vi "SetTilesTMX.vi"(8 "error in (no error)":errorcluster, 9 "Position":T1, 10 "path to tmx-file (created with Tiles2D)":path=path "/home/lvuser/natinst/bin/data/maps/Menu.tmx", 11 "Game in":refnum<class "Game.lvclass">) -> (0 "error out":errorcluster, 3 "Game out":refnum<class "Game.lvclass">)   [LabVIEW 2019, in "RT_Game.lvlib" / "Game.lvclass"]
uses:
  Game.lvclass
  Coordinate.ctl
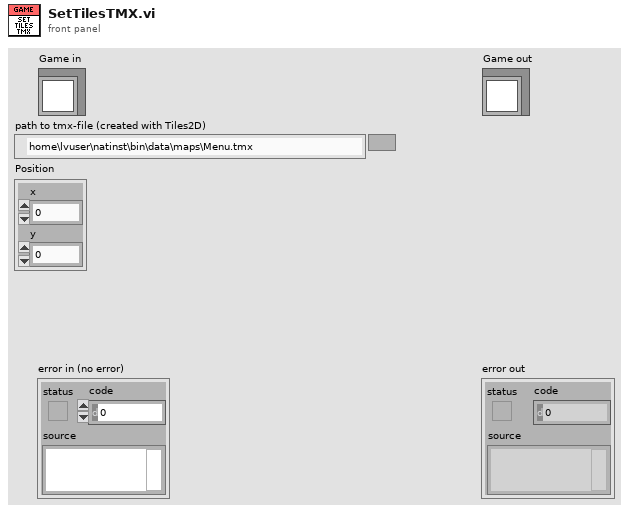
[diagram p1: front panel]
types:
  T1 = typedef "RT_Game.lvlib/Game.lvclass/Coordinate.ctl" = cluster{"x":dbl, "y":dbl}
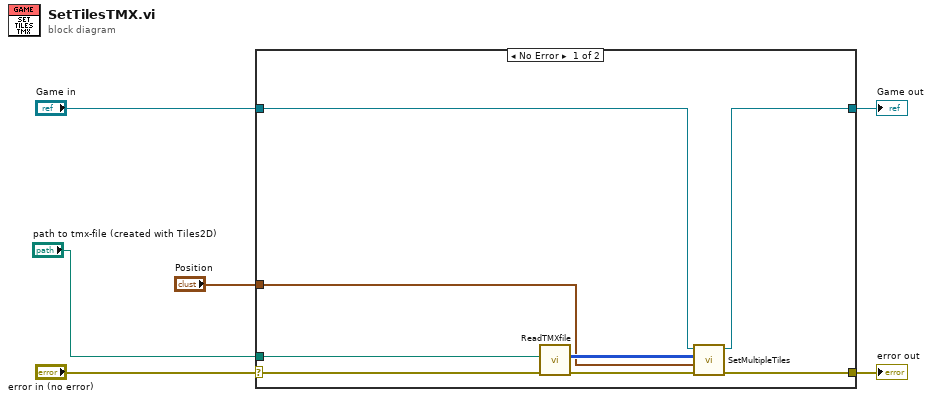
[diagram p0: block diagram]
diagram:
  n1 = case shown="No Error" "error in (no error)" {
    selector: "error in (no error)" -> [w14 w16]
    tunnel: [w11 w16] -> w5
    tunnel: [w10 w15] -> w3
    tunnel: "Game in" -> [w9 w15]
    tunnel: "path to tmx-file (created with Tiles2D)" -> [w12 _]
    tunnel: "Position" -> [w7 _]
    frame No Error {
      n2 = call "ReadTMXfile.vi"("error in (no error)"=w14, "path to tmx-file (created with Tiles2D)"=w12) -> ("error out"=w13:errorcluster, "Tilenumbers"=w8:u32[][])  [unwired: 8 in]
      n3 = call "SetMultipleTiles.vi"("error in (no error)"=w13, "Position"=w7, "TileCodes"=w8, "Game in"=w9) -> ("error out"=w11:errorcluster, "Game out"=w10:refnum<class "Game.lvclass">)  [unwired: 6 in]
    }
    frame Error {
    }
  }
  "error out" <- w5
  "Game out" <- w3
